vi "logbook.vi"() -> ()   [LabVIEW 2017]
uses:
  <vilib>/sound2/lvsound2.llb/Sound Data Format.ctl
  <vilib>/sound2/lvsound2.llb/Sampling Mode.ctl
  globalUtilities.vi
  <vilib>/sound2/lvsound2.llb/Sound File Write Open.vi
  <vilib>/sound2/lvsound2.llb/Sound Input Read (DBL).vi
  <vilib>/sound2/lvsound2.llb/Sound File Write (DBL).vi
panel:
  out "Log book path":string
  out "Last audio saved":string
  out "recording":bool
  in  "STOP PROGRAM":bool
  in  "Stop audio recording":bool
  in  "Start audio recording":bool
  out "folderPresent":bool
  in  "Save entry":bool
  in  "Log book entry":string
  # "LOG BOOK"
  # "TEXT ENTRIES TO LOG BOOK"
  # "AUDIO ENTRIES TO LOG BOOK"
  # "The log book will have a text entry with the filename of the\ncorresponding audio file."
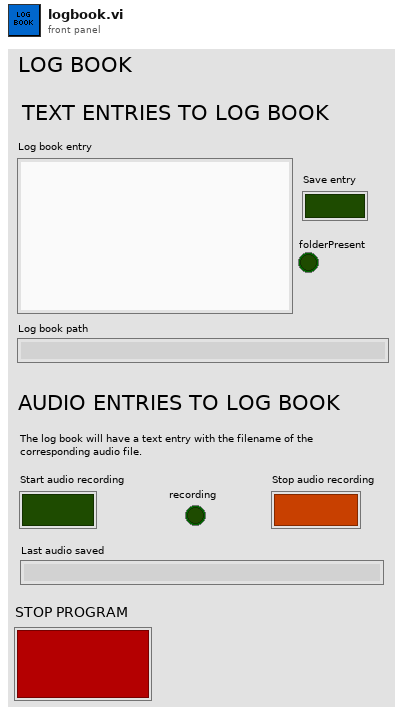
[diagram p1: front panel]
types:
  T1 = typedef "Sound Data Format.ctl" = cluster{"sample rate (S/s)":dbl, "number of channels":i32, "bits per sample":i32}
  T2 = typedef "Sampling Mode.ctl" = i32
  T3 = typedef "Sound Input Task ID.ctl" = u32
  T4 = typedef "Sound File Refnum.ctl" = refnum<file>
  T5 = cluster{"button info":cluster{"button 1":bool, "button 2":bool, "button 3":bool, "button 4":bool, "button 5":bool, "button 6":bool, "button 7":bool, "button 8":bool, "button 9":bool, "button 10":bool, "button 11":bool, "button 12":bool, "button 13":bool, "button 14":bool, "button 15":bool, "button 16":bool, "button 17":bool, "button 18":bool, "button 19":bool, "button 20":bool, "button 21":bool, "button 22":bool, "button 23":bool, "button 24":bool, "button 25":bool, "button 26":bool, "button 27":bool, "button 28":bool, "button 29":bool, "button 30":bool, "button 31":bool, "button 32":bool}, "direction info":cluster{"pov 1":i32, "pov 2":i32, "pov 3":i32, "pov 4":i32}, "axis info":cluster{"X axis":i32, "Y axis":i32, "Z axis":i32, "X axis rotation":i32, "Y axis rotation":i32, "Z axis rotation":i32, "U axis":i32, "V axis":i32}}
  T6 = cluster{"X axis":i32, "Y axis":i32, "Z axis":i32, "X axis rotation":i32, "Y axis rotation":i32, "Z axis rotation":i32, "U axis":i32, "V axis":i32}
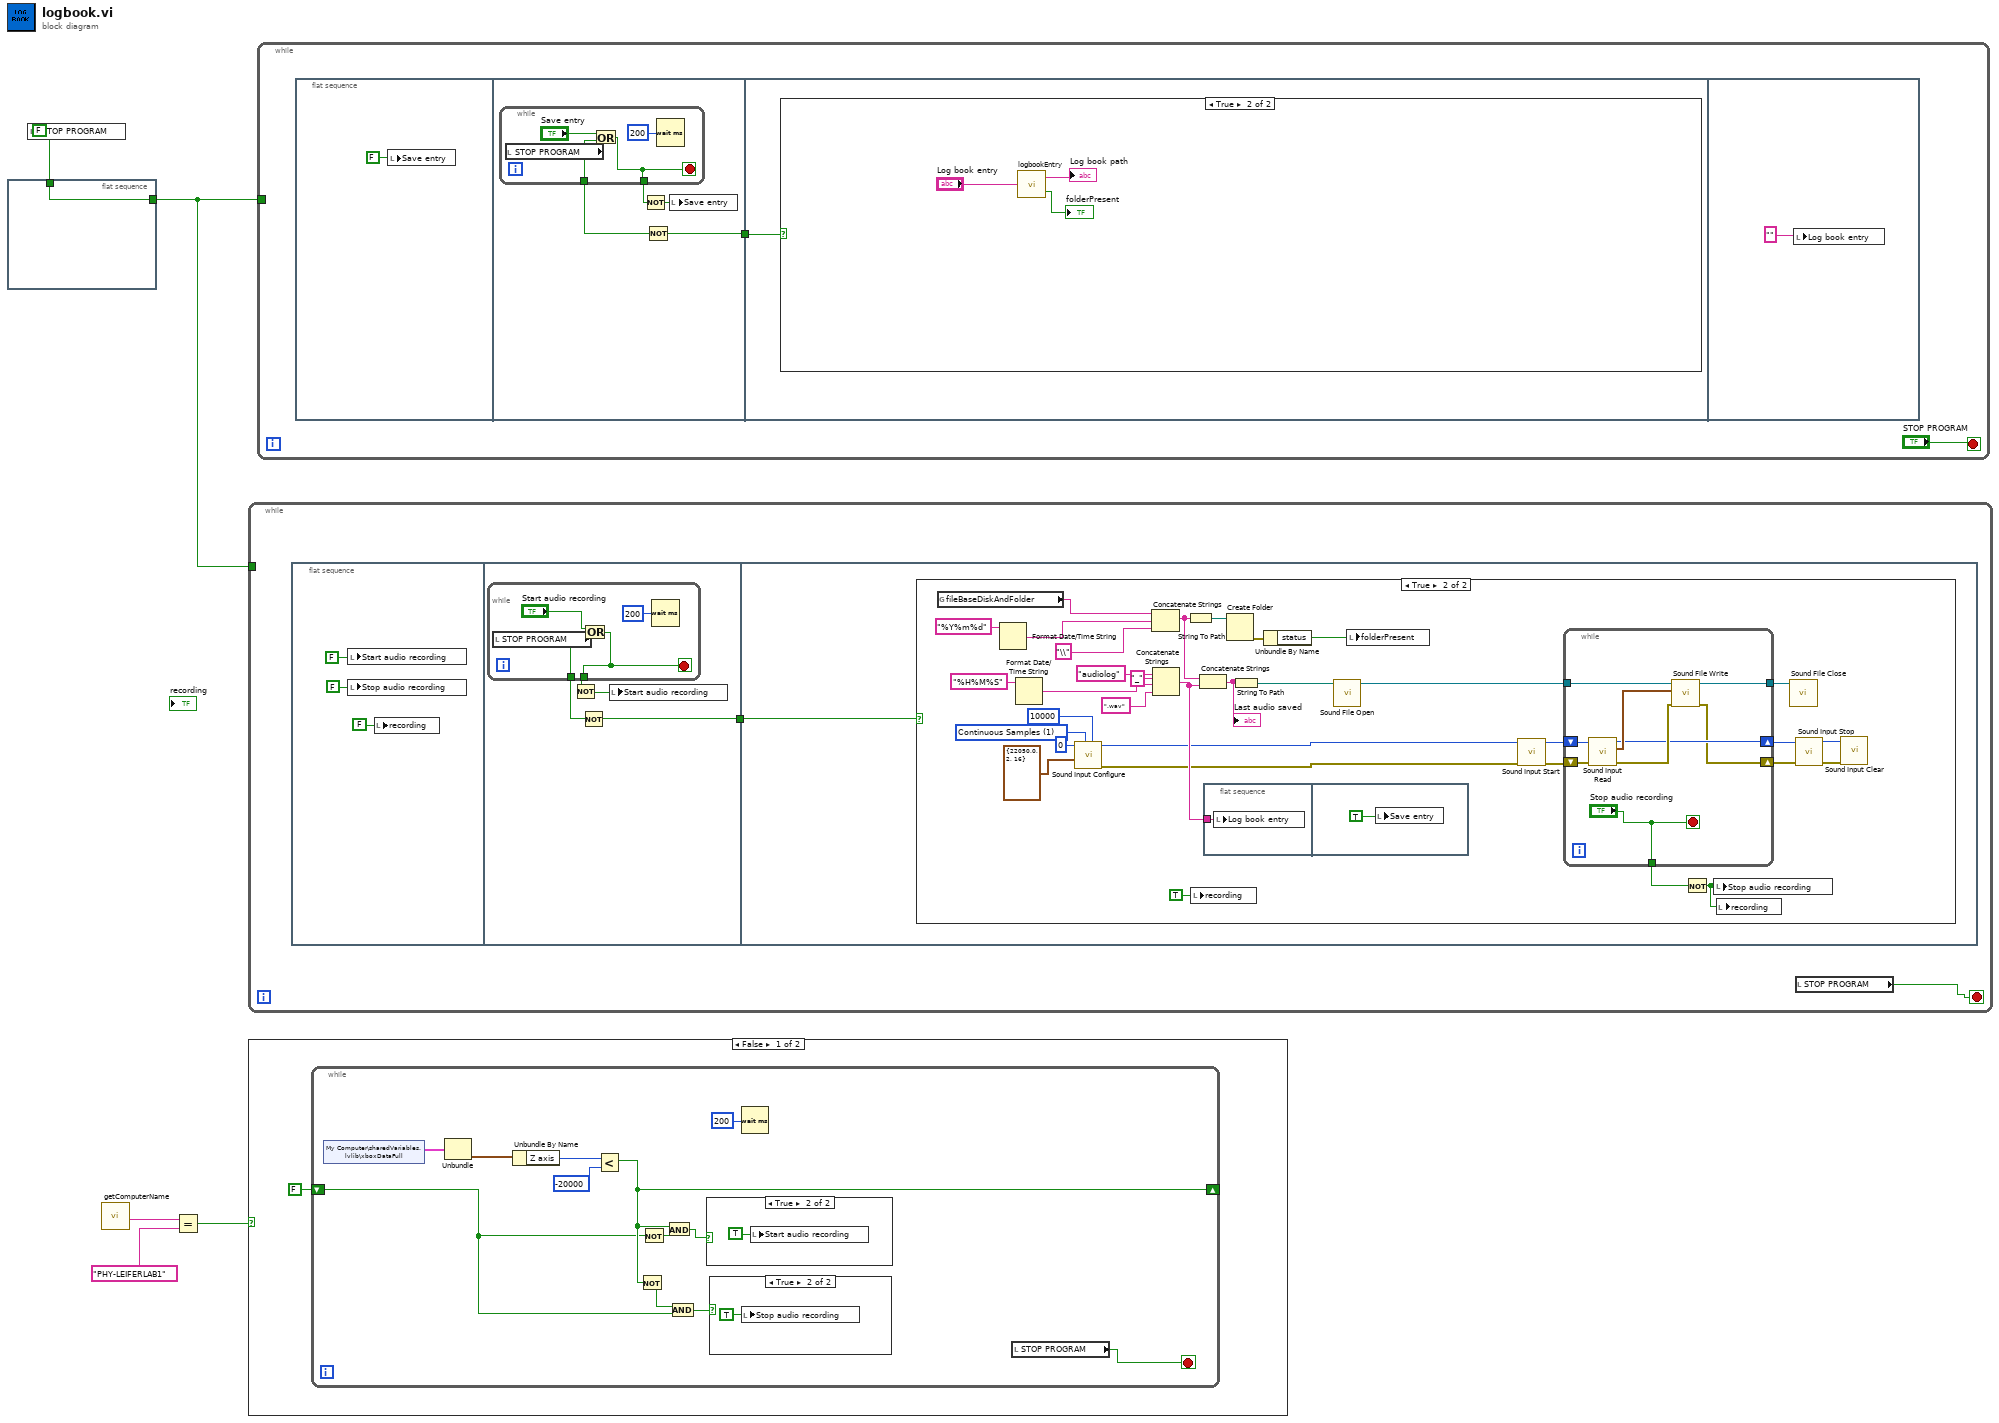
[diagram p0: block diagram]
diagram:
  w5 = FALSE ("STOP")
  n1 = flat-sequence {
    tunnel: w5 -> [w6]
    tunnel: [w6] -> w4
    frame #0 {
    }
  }
  n2 = local write "STOP PROGRAM"(w5) -> ()
  n3 = call "getComputerName.vi"() -> ("name"=w3:string)  [unwired: 1 in, 2 out]
  n4 = Equal?(x=w3, y="PHY-LEIFERLAB1") -> (x = y?=w2:bool)
  n5 = while {
    tunnel: w4 -> [_]
    stop <- w7 stop-if-true
    n6 = flat-sequence {
      tunnel: [w13] -> w8
      tunnel: w8 -> [w20]
      frame #0 {
        n7 = local write "Start audio recording"(FALSE ("Record audio")) -> ()
        n8 = local write "Stop audio recording"(FALSE ("Start audio recording")) -> ()
        n9 = local write "recording"(FALSE ("recording")) -> ()
      }
      frame #1 {
        n10 = while {
          tunnel: [w18] -> w15
          tunnel: [w17] -> w14
          stop <- w18 stop-if-true
          n11 = local read "STOP PROGRAM"() -> (w17:bool)
          n12 = Or(x="Start audio recording", y=w17) -> (x .or. y?=w18:bool)
          n13 = Wait (ms)(milliseconds to wait=u32 200) -> ()  [unwired: 1 out]
        }
        n14 = Not(x=w15) -> (.not. x?=w12:bool)
        n15 = Not(x=w14) -> (.not. x?=w13:bool)
        n16 = local write "Start audio recording"(w12) -> ()
      }
      frame #2 {
        n17 = case shown="True" w20 {
          frame False {
          }
          frame True {
            w31 = T2 1 items=["Finite Samples", "Continuous Samples"] ("sample mode")
            n18 = global read "globalUtilities.vi" "fileBaseDiskAndFolder"() -> (w45:string)
            n19 = Format Date/Time String(time format string (%c)="%Y%m%d") -> (date/time string=w44:string)  [unwired: 2 in]
            n20 = Format Date/Time String(time format string (%c)="%H%M%S") -> (date/time string=w43:string)  [unwired: 2 in]
            n21 = call <vilib>:"Sound Input Configure.vi"("number of samples/ch"=10000, "sample mode"=w31, "sound format"=T1 {"sample rate (S/s)"=22050.0, "number of channels"=2, "bits per sample"=16}, "device ID"=u32 0) -> ("error out"=w25:errorcluster, "task ID"=w28:T3)  [unwired: 6 in]
            n22 = Concatenate Strings(w45, w44, "\\") -> (w39:string)
            n23 = Concatenate Strings("audiolog" ("string"), "_" ("string"), w43, ".wav" ("string")) -> (w38:string)
            n24 = String To Path(string=w39) -> (path=w46:path)
            n25 = local write "recording"(TRUE ("recording")) -> ()
            n26 = Concatenate Strings(w39, w38) -> (w40:string)
            "Last audio saved" <- w40
            n27 = flat-sequence {
              tunnel: w38 -> [w54]
              frame #0 {
                n28 = local write "Log book entry"(w54) -> ()
              }
              frame #1 {
                n29 = local write "Save entry"(TRUE) -> ()
              }
            }
            n30 = Create Folder(path (use dialog)=w46) -> (error out=w47:errorcluster)  [unwired: 2 in, 2 out]
            n31 = String To Path(string=w40) -> (path=w41:path)
            n32 = Unbundle By Name(w47) -> ("status"=w42:bool)
            n33 = call-poly <vilib>:"Sound File Open.vi"("path"=w41) -> ("sound file refnum"=w33:T4)  [unwired: 9 in, 1 out]
            n34 = local write "folderPresent"(w42) -> ()
            n35 = call <vilib>:"Sound Input Start.vi"("error in (no error)"=w25, "task ID"=w28) -> ("error out"=w52:errorcluster, "task ID out"=w53:T3)  [unwired: 8 in]
            n36 = while {
              shift-right: [w58] -> w50
              shift-left: w52 -> [w63]
              shift-right: [w60] -> w49
              shift-left: w53 -> [w64]
              tunnel: [w59] -> w51
              tunnel: ["Stop audio recording"] -> w48
              tunnel: w33 -> [w56]
              stop <- "Stop audio recording" stop-if-true
              n37 = call-poly <vilib>:"Sound Input Read.vi"("error in (no error)"=w63, "task ID"=w64) -> ("error out"=w61:errorcluster, "data"=w62:waveform(dbl)[], "task ID out"=w60:T3)  [unwired: 7 in]
              n38 = call-poly <vilib>:"Sound File Write.vi"("error in (no error)"=w61, "data"=w62, "sound file refnum"=w56) -> ("error out"=w58:errorcluster, "sound file refnum out"=w59:T4)  [unwired: 7 in]
            }
            n39 = Not(x=w48) -> (.not. x?=w23:bool)
            n40 = local write "Stop audio recording"(w23) -> ()
            n41 = local write "recording"(w23) -> ()
            n42 = call <vilib>:"Sound File Close.vi"("sound file refnum"=w51) -> ()  [unwired: 10 in, 1 out]
            n43 = call <vilib>:"Sound Input Stop.vi"("error in (no error)"=w50, "task ID"=w49) -> ("error out"=w26:errorcluster, "task ID out"=w27:T3)  [unwired: 8 in]
            n44 = call <vilib>:"Sound Input Clear.vi"("error in (no error)"=w26, "task ID"=w27) -> ()  [unwired: 9 in, 1 out]
          }
        }
      }
    }
    n45 = local read "STOP PROGRAM"() -> (w7:bool)
  }
  n46 = case shown="False" w2 {
    frame False {
      n47 = while {
        shift-right: [w71] -> _
        shift-left: FALSE -> [w69]
        stop <- w73 stop-if-true
        n48 = shared-variable "My Computer\\sharedVariables.lvlib\\xboxDataFull"() -> (w77:T5)  [unwired: 1 in, 1 out]
        n49 = Unbundle(w77) -> ("axis info"=w76:T6)  [unwired: 2 out]
        n50 = Unbundle By Name(w76) -> ("Z axis"=w75:i32)
        n51 = Less?(x=w75, y=-20000) -> (x < y?=w71:bool)
        n52 = Not(x=w71) -> (.not. x?=w72:bool)
        n53 = Not(x=w69) -> (.not. x?=w70:bool)
        n54 = And(x=w71, y=w70) -> (x .and. y?=w68:bool)
        n55 = And(x=w72, y=w69) -> (x .and. y?=w67:bool)
        n56 = case shown="True" w68 {
          frame False {
          }
          frame True {
            n57 = local write "Start audio recording"(TRUE ("Start audio recording")) -> ()
          }
        }
        n58 = case shown="True" w67 {
          frame False {
          }
          frame True {
            n59 = local write "Stop audio recording"(TRUE ("Stop audio recording")) -> ()
          }
        }
        n60 = Wait (ms)(milliseconds to wait=u32 200) -> ()  [unwired: 1 out]
        n61 = local read "STOP PROGRAM"() -> (w73:bool)
      }
    }
    frame True {
    }
  }
  n62 = while {
    tunnel: w4 -> [_]
    stop <- "STOP PROGRAM" stop-if-true
    n63 = flat-sequence {
      tunnel: [w83] -> w81
      tunnel: w81 -> [w91]
      frame #0 {
        n64 = local write "Save entry"(FALSE ("Save entry")) -> ()
      }
      frame #1 {
        n65 = while {
          tunnel: [w90] -> w86
          tunnel: [w88] -> w84
          stop <- w90 stop-if-true
          n66 = local read "STOP PROGRAM"() -> (w88:bool)
          n67 = Or(x="Save entry", y=w88) -> (x .or. y?=w90:bool)
          n68 = Wait (ms)(milliseconds to wait=u32 200) -> ()  [unwired: 1 out]
        }
        n69 = Not(x=w86) -> (.not. x?=w85:bool)
        n70 = Not(x=w84) -> (.not. x?=w83:bool)
        n71 = local write "Save entry"(w85) -> ()
      }
      frame #2 {
        n72 = case shown="True" w91 {
          frame False {
          }
          frame True {
            n73 = call "logbookEntry.vi"("Log book entry"="Log book entry") -> ("Log book path"=→"Log book path":string, "folderPresent"=→"folderPresent":bool)
          }
        }
      }
      frame #3 {
        n74 = local write "Log book entry"("" ("Log book entry")) -> ()
      }
    }
  }
